vi "Digital Write.vi"(8 "Error In":errorcluster, 9 "Values":bool[](array[boolean]), 10 "Channels":u8[](array[numeric]), 11 "LINX Device Config":T1) -> (0 "Error Out":errorcluster, 3 "LINX Device Config":T1)   [LabVIEW 2020, in "Device.lvlib"]
doc: "Set the value of one or more digital output pin."
uses:
  Device.lvlib
  Type Defs/LINX Device Config.ctl
  Type Defs/Interface.ctl
  Type Defs/TCP Config.ctl
  Type Defs/Channels.ctl
  Type Defs/Error Type.ctl
  LMH-LINX.lvlib
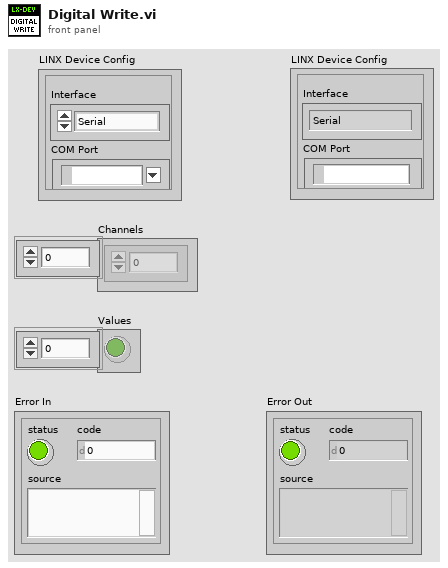
[diagram p1: front panel]
types:
  T1 = typedef "Device.lvlib/LINX Device Config.ctl" = cluster{"Interface":T2, "COM Port":refnum<visa-resource-name>, "TCP Configuration":T3, "Device Family":u8, "Device ID":u8, "Device Name":string, "TCP Ref":refnum<k5>, "Channels":T4}
  T2 = typedef "LMH-LINX.lvlib/Interface.ctl" = enum16{"Serial", "TCP"}
  T3 = typedef "Device.lvlib/TCP Config.ctl" = cluster{"IP Address":string, "Port":u16}
  T4 = typedef "LMH-LINX.lvlib/Channels.ctl" = cluster{"DI":u8[], "DO":u8[], "AI":u8[], "AO":u8[], "PWM":u8[], "QE":u8[], "UART":u8[], "I2C 2":u8[], "SPI":u8[], "CAN":u8[], "Servo":u8[], "AI Ref (V)":dbl, "AI Resolution (Bits)":u8, "AO Ref (V)":dbl, "AO Resolution (Bits)":u8}
  T5 = typedef "LMH-LINX.lvlib/Error Type.ctl" = enum16{"Unknown", "Timeout", "Corrupt Return Packet", "Unable To Connect", "Command Not Supported", "Channel DNE", "Invalid COM Config", "Firmware Version Mismatch", "myRIO Support", "CMD Specific Error", "Local IO Not Supported"}
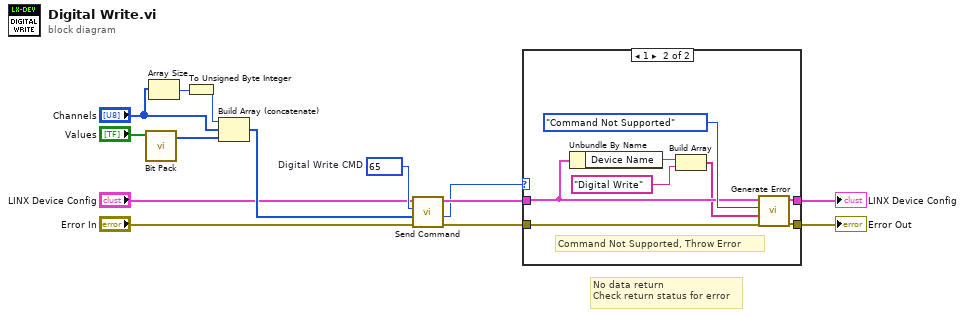
[diagram p0: block diagram]
diagram:
  w13 = u16 65  # Digital Write CMD
  # "No data return\nCheck return status for error"
  n1 = call "Bit Pack.vi"("Values"="Values") -> ("Packed Values"=w9:u8[])  [unwired: 10 in]
  n2 = Array Size(array="Channels") -> (size(s)=w12:i32)
  n3 = To Unsigned Byte Integer(number=w12) -> (unsigned 8bit integer=w11:u8)
  n4 = Build Array (concatenate)(w11, "Channels", w9) -> (w10:u8[])
  n5 = call "Send Command.vi"("Error In"="Error In", "ARGS"=w10, "CMD"=w13, "LINX Device Config"="LINX Device Config") -> ("Error Out"=w6:errorcluster, "Status"=w1:u8, "LINX Device Config"=w4:T1)  [unwired: 4 in, 1 out]
  n6 = case shown="1" w1 {
    tunnel: [w16 w22] -> w8
    tunnel: w4 -> [w16 w18]
    tunnel: [w15 w23] -> w7
    tunnel: w6 -> [w15 w24]
    frame 0, Default {
      # "Status OK"
    }
    frame 1 {
      # "Command Not Supported, Throw Error"
      n7 = Unbundle By Name(w18) -> ("Device Name"=w20:string)
      n8 = Build Array(w20, "Digital Write") -> (w17:string[])
      n9 = call "Generate Error.vi"("Error In"=w24, "Arguments"=w17, "Error Type"=Error_Type."Command Not Supported", "LINX Device Config"=w18) -> ("Error Out"=w23:errorcluster, "Dup LINX Device Config"=w22:T1)  [unwired: 6 in]
    }
  }
  "Error Out" <- w7
  "LINX Device Config" <- w8
